vi "TimeTaskerVr4.vi"(0 "Delay(sec)":dbl, 1 "Start Counting?":bool) -> (2 "TimePast?":bool, 3 "TimePast":dbl, 4 "Counting?":bool)   [LabVIEW 2012]
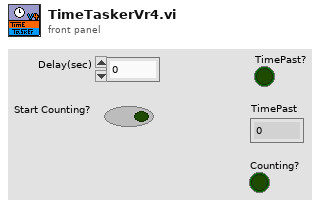
[diagram p1: front panel]
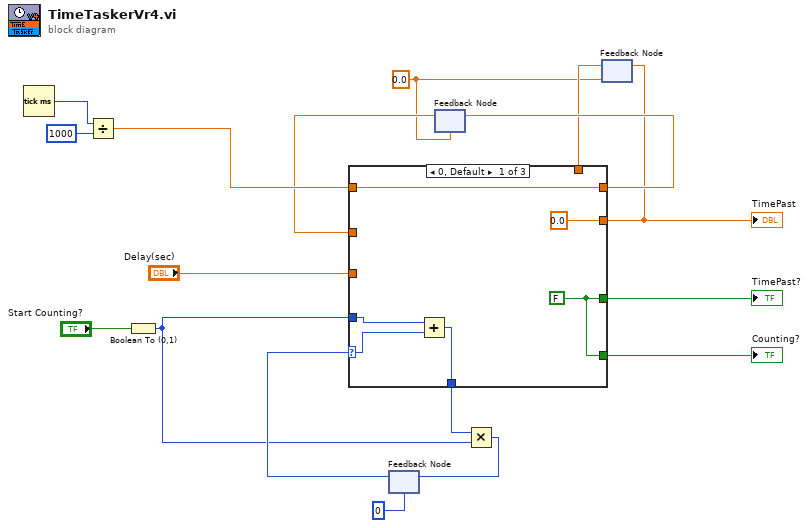
[diagram p0: block diagram]
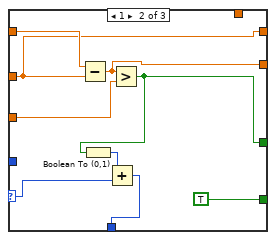
[diagram p2: hidden frame]
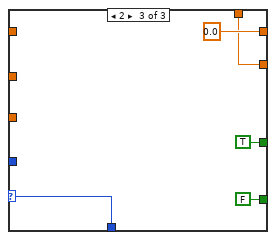
[diagram p3: hidden frame]
diagram:
  w7 = 0.0 ("f")
  n1 = Tick Count (ms)() -> (millisecond timer value=w16:u32)
  n2 = Divide(x=w16, y=u32 1000) -> (x/y=w14:dbl)
  n3 = Boolean To (0,1)(Boolean="Start Counting?") -> (0, 1=w1:i16)
  n4 = feedback #1(i16 0 ("0, 1")) -> (w5:i16)
  n5 = feedback #2(w7) -> (w12:dbl)
  n6 = feedback #3(w7) -> (w9:dbl)
  n7 = case shown="0, Default" w5 {
    selector: w5 -> [w20 w25 w33]
    tunnel: [0.0 w29 w36] -> w8
    tunnel: [w23 w27 TRUE ("Counting?")] -> w10
    tunnel: [w23 TRUE ("Counting?") FALSE ("Counting?")] -> w15
    tunnel: w14 -> [w21 w31 _]
    tunnel: [w21 w30 0.0 ("f")] -> w13
    tunnel: w12 -> [_ w30 _]
    tunnel: "Delay(sec)" -> [_ w28 _]
    tunnel: w9 -> [_ _ w36]
    tunnel: w1 -> [w19 _ _]
    tunnel: [w18 w24 w33] -> w3
    frame 0, Default {
      w23 = FALSE ("Counting?")
      n8 = Add(x=w19, y=w20) -> (x+y=w18:i16)
    }
    frame 1 {
      n9 = Subtract(x=w31, y=w30) -> (x-y=w29:dbl)
      n10 = Greater?(x=w29, y=w28) -> (0:w27:bool)
      n11 = Boolean To (0,1)(Boolean=w27) -> (0, 1=w26:i16)
      n12 = Add(x=w26, y=w25) -> (x+y=w24:i16)
    }
    frame 2 {
    }
  }
  "TimePast?" <- w10
  "Counting?" <- w15
  "TimePast" <- w8
  n13 = feedback-in #2(w13) -> ()
  n14 = Multiply(x=w3, y=w1) -> (x*y=w2:i16)
  n15 = feedback-in #1(w2) -> ()
  n16 = feedback-in #3(w8) -> ()
